vi "Theme Editor Config--constant.vi"() -> (3 "Button Editor Config":path)   [LabVIEW 2021, in "Theme Config.lvclass"]
doc: "Constant VI to define the location of the theme editor configuration file.\n\n<b>Code Developed By:</b> +\nDaniel Coons +\nTechnology Service Corporation +\nwww.tsc.com/atcs"
uses:
  Theme Config.lvclass
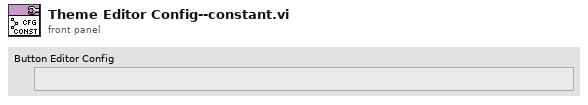
[diagram p1: front panel]
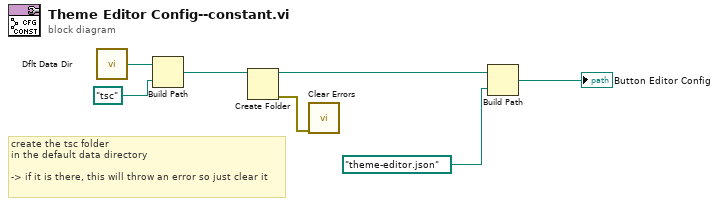
[diagram p0: block diagram]
diagram:
  # "create the tsc folder\nin the default data directory\n\n-> if it is there, this will throw an error so just clear it"
  n1 = call <vilib>:"Dflt Data Dir.vi"() -> ("App:Default Data Directory"=w4:path)
  n2 = Build Path(base path=w4, name or relative path=path "tsc") -> (appended path=w6:path)
  n3 = Create Folder(path (use dialog)=w6) -> (created path=w2:path, error out=w7:errorcluster)  [unwired: 2 in, 1 out]
  n4 = call <vilib>:"Clear Errors.vi"("error in (no error)"=w7) -> ()  [unwired: 5 in, 2 out]
  n5 = Build Path(base path=w2, name or relative path=path "theme-editor.json") -> (appended path=→"Button Editor Config":path)
